vi "instrumentProperties_spectrometerIndex.vi"(8 "error in (no error)":errorcluster, 11 "Thorlabs_OSA_64 in":refnum<class "OSA.lvclass">) -> (0 "error out":errorcluster, 2 "spectrometerIdx":u16, 3 "Thorlabs_OSA_64 out":refnum<class "OSA.lvclass">)   [LabVIEW 2010, in "OSA.lvclass"]
uses:
  OSA.lvclass
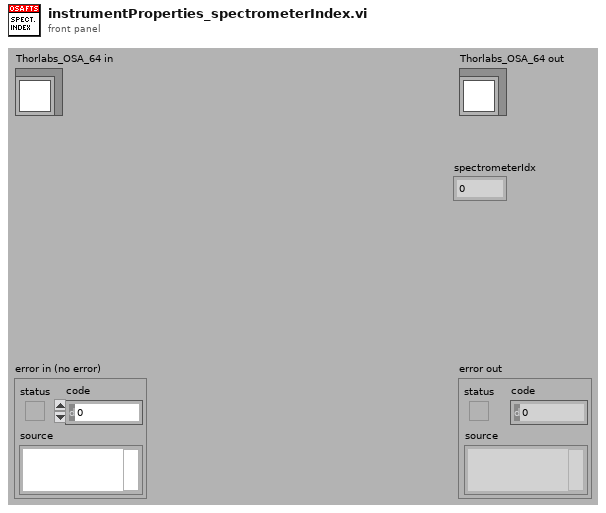
[diagram p1: front panel]
types:
  T1 = typedef "OSA.lvclass/ObjectAttributes.ctl" = cluster{"Stop":bool, "dataType":T2, "spectrometerIdx":u16, "buffer size interferogram":i32, "interferogram":cluster{"new":bool, "plot_x_ min":sgl, "plot_x_max":sgl, "plot_y_min":sgl, "plot_y_max":sgl, "Graph Intrfrgrm":T3, "timeStamp":u32, "signal (%)":dbl, "traces":cluster{"idx":u32, "broadBand":bool, "monoChromatic":bool, "peakToPeakSignal":dbl, "peakToPeakPos":dbl}[], "traces idx last":i32, "contrast (%)":dbl}, "spectrum":cluster{"new":bool, "plot_x_min":sgl, "plot_x_max":sgl, "plot_unit_x":T4, "plot_unit_y":T5, "plot_y_min":sgl, "plot_y_max":sgl, "Graph Spectrum":T3, "timeStamp":u32, "X_VAL_OPTIONS":enum16{"MIN_MAX", "ARRAY"}, "traces":cluster{"idx":u32}[], "traces idx last":i32}, "Thorlabs_OSA_64.lvclass:queue_action.ctlqueue ref":refnum<queue>, "action":T6, "plot zoom step":dbl, "buffer semaphore":T7, "acq stopped":bool, "dataType active":T2, "temperature (degr C)":sgl, "pressure (hPa)":sgl, "rel humidity (%)":sgl, "settings":cluster{"resolution":u16, "sensitivity":u16, "Average":bool, "average nr":u32, "apodisation":T8, "acq delay (ms)":u32, "airMesure":T9, "wmtr on":bool, "intfgrm_smooth_width":u16, "intfgrm_smooth_nrOfPasses":u16, "intfgrm_smooth":T10, "phaseCorrection":T11, "zeroFill":u8, "spectr_smooth":T10, "spectr_smooth_width":u16, "spectr_smooth_nrOfPasses":u16, "resolution (/cm)":sgl, "REF wavelength, (nm)":dbl, "gain_idx":u16, "gainAuto":bool, "gain_relative":dbl, "PD sensitivity mode":T12, "PD senseMode implemented":bool, "SensorTemperature implemented":bool, "SensorPressure implemented":bool, "SensorHumidity implemented":bool, "attenuationAuto":bool, "attenuationOnOff":bool, "attenuationAvailable":bool, "offsetAvailable":bool, "offset":i32, "offset max":u16, "contrastAvailable":bool}, "peaks position":sgl[], "peaks width":sgl[], "peaks height":sgl[], "peaks max nr":u32, "peaks latest nr":i32, "peaks new":bool, "power":dbl, "power new":bool, "path":string, "wavelength (WNr)":dbl, "wavelength new":bool, "buffer size spectrum":i32, "status":string, "vi reference":refnum<vi>, "funcPointer":u64, "libraryPointer":u64, "singleAcquisition":bool, "coherenceLength (cm)":dbl, "coherenceLength new":bool, "spectrometer model":string, "spectrometer serial nr":string, "peaks thld left":sgl[], "peaks thld right":sgl[], "coherenceLength error (cm)":dbl, "ADC bits":u16, "peaks position centroid":sgl[], "peaks height centroid":sgl[], "OSA series":T13, "channel index spectrum":u16, "spectrometer rangeLow, (/cm)":dbl, "spectrometer rangeHigh, (/cm)":dbl, "channel index interferogram":u16, "virtualSource":bool, "sweep restart":bool}
  T2 = typedef "OSA.lvclass/acq_dataType.ctl" = enum16{"none", "interferogram", "spectrum"}
  T3 = typedef "OSA.lvclass/graph_intensity.ctl" = refnum<vi>
  T4 = typedef "OSA.lvclass/spectrum_x_unit.ctl" = enum16{"wavenr/cm", "THz", "eV", "nm_air", "nm_vac"}
  T5 = typedef "OSA.lvclass/y_unit.ctl" = enum16{"ADC counts", "dBm pwr absolute", "dBm pwr density", "mW pwr absolute", "mW pwr density"}
  T6 = typedef "OSA.lvclass/queue_action.ctl" = enum16{"none", "stop", "GUI_plotInterferogram", "GUI_plotSpectrum", "GUI_plotInterferogramRescale", "GUI_plotSpectrumRescale", "GUI_plotInterferogramReset", "GUI_plotSpectrumReset", "GUI_plotInterferogramAutoScaleY", "GUI_plotSpectrumAutoScaleY", "GUI_plotInterferogramZoomOut", "GUI_plotSpectrumZoomOut", "GUI_plotInterferogramPane", "GUI_plotSpectrumPane", "GUI_plotInterferogramZoomMouse", "GUI_plotSpectrumZoomMouse", "GUI_plotSpectrumFSRY", "GUI_plotInterferogramFSRY", "GUI_spectrumChannelType", "GUI_channel", "ENVIRONMENT temperature", "ENVIRONMENT pressure", "MODE_resolution set", "MODE_resolution get", "MODE_sensitivity set", "MODE_sensitivity get", "MODE_PDTemperature set", "MODE_PDTemperature get", "REBOOT/RESET firmware", "ACQASYNC_acquireSingleSpectrum", "ACQASYNC_continuous start", "ACQASYNC_continuous stop\n", "ACQASYNC_get last interferogram", "ACQASYNC_get last spectrum", "ACQASYNC_get last waveNr", "ACQOPT_interferogram smoothing set", "ACQOPT_interferogram smoothing get", "ACQOPT_spectrum smoothing set", "ACQOPT_spectrum smoothing get", "ACQOPT_apodisation type set", "ACQOPT_apodisation type get", "ACQOPT_phase correction type set", "ACQOPT_phase correction type get", "ACQOPT_acqIntervall_set", "ACQOPT_acqIntervall_get", "ACQOPT_average spectrum set", "ACQOPT_average spectrum get", "ACQOPT_rolling average set", "ACQOPT_rolling average get", "ACQOPT_zero fill factor set", "ACQOPT_zero fill factor get", "ACQOPT_cycle counting set", "ACQOPT_cycle counting get", "ACQOPT_air measure option set", "ACQOPT_air measure option get", "ACQOPT_gainLevel auto get", "ACQOPT_gainLevel auto set", "ACQOPT_gainLevel get", "ACQOPT_gainLevel set", "ACQOPT_offset set", "ACQOPT_attenuator_auto_set", "ACQOPT_attenuator_set", "ACQOPT_getAll", "INSTRUMENT_PROPERTY_range_WaveNr_min", "INSTRUMENT_PROPERTY_range_WaveNr_max", "INSTRUMENT_PROPERTY_reference_wavelength_cm^-1", "INSTRUMENT_PROPERTY_samplesPerRefPeriod", "INSTRUMENT_PROPERTY_resolution_waveNrPercm", "INSTRUMENT_PROPERTY_availableGainLevels", "INSTRUMENT_PROPERTY_status", "CONVERT", "ANALYSE_POWER", "ANALYSE_PEAKS", "ANALYSE_WAVELENGTH", "ANALYSE_SPECTRUM", "ANALYSE_INTERFEROGRAM", "ANALYSE_COHERENCE_LENGTH", "MATH", "MATH_power", "MATH_peaks", "FILE", "miscellaneous"}
  T7 = typedef "Semaphore RefNum" = refnum<k1>
  T8 = typedef "OSA.lvclass/apodisation.ctl" = enum16{"NONE", "NORTON_BEER_WEAK", "NORTON_BEER_MEDIUM", "NORTON_BEER_STRONG", "TRIANGULAR", "COSINE", "HANN", "HAMMING", "BLACKMANHARRIS3", "BLACKMANHARRIS4", "GAUSSIAN"}
  T9 = typedef "OSA.lvclass/airMeasure.ctl" = enum16{"TEMPERATURE", "PRESSURE"}
  T10 = typedef "OSA20X_misc.lvlib/interferogram_smoothing.ctl" = enum16{"NONE", "BINOMIAL", "SAVITSKY_GOLAY", "FOURIER", "MOVING_AVERAGE", "GAUSSIAN"}
  T11 = typedef "OSA.lvclass/phaseCorrection.ctl" = enum16{"NONE", "MERTZ", "FORMAN", "MERTZ_FILE", "FORMAN_FILE", "FUTURE COMP."}
  T12 = typedef "OSA20X_misc.lvlib/PDTemperatureMode.ctl" = enum16{"cool: better sensitivity/noise floor", "warm: extended wl range"}
  T13 = typedef "OSA.lvclass/OSA_series.ctl" = enum16{"OSA200", "OSA300", "UNKNOWN"}
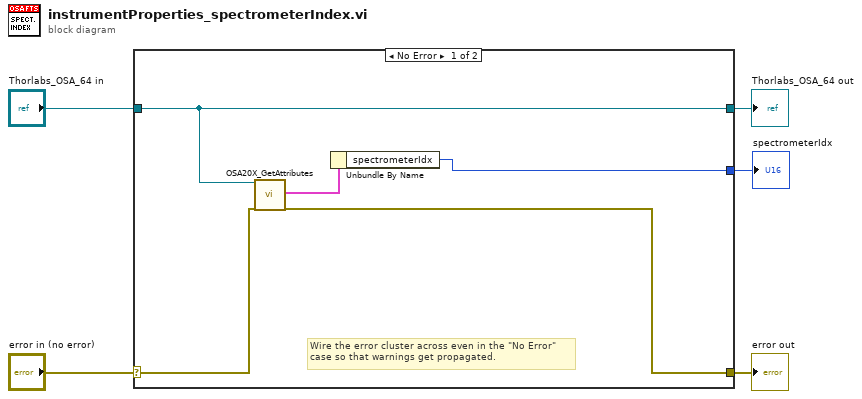
[diagram p0: block diagram]
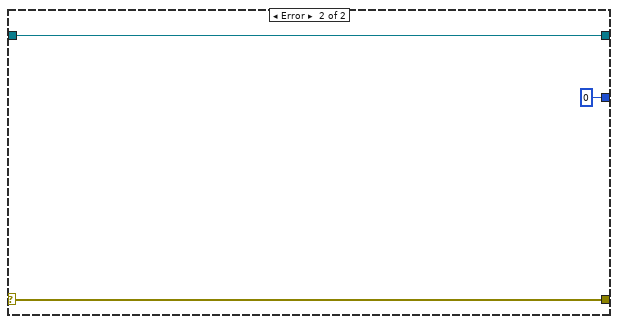
[diagram p2: hidden frame]
diagram:
  n1 = case shown="No Error" "error in (no error)" {
    selector: "error in (no error)" -> [w8 w13]
    tunnel: [w7 w13] -> w4
    tunnel: [w9 w12] -> w2
    tunnel: "Thorlabs_OSA_64 in" -> [w9 w12]
    tunnel: [w6 u16 0 ("spectrometerIdx")] -> w1
    frame No Error {
      # "Wire the error cluster across even in the \"No Error\"\ncase so that warnings get propagated."
      n2 = call "OSA20X_GetAttributes.vi"("reference in"=w9, "error in (no error)"=w8) -> ("Data"=w10:T1, "error out"=w7:errorcluster)  [unwired: 14 in, 2 out]
      n3 = Unbundle By Name(w10) -> ("spectrometerIdx"=w6:u16)
    }
    frame Error {
    }
  }
  "error out" <- w4
  "Thorlabs_OSA_64 out" <- w2
  "spectrometerIdx" <- w1
